vi "TTM 4He Press to Temp.vi"(1 "4He Vapor Pressure (torr)":dbl format="%.3f") -> (0 "4He Temp (K)":dbl format="%.3f")   [LabVIEW 2019]
panel:
  # "ITS-90 valid only from 1.25K to 2.17K"
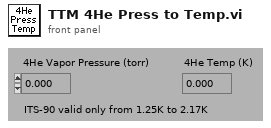
[diagram p1: front panel]
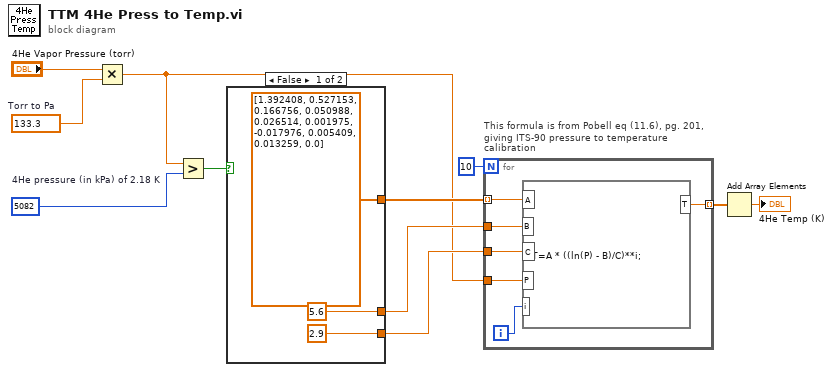
[diagram p0: block diagram]
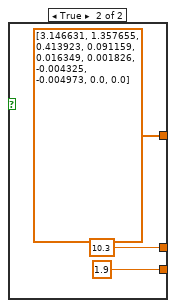
[diagram p2: hidden frame]
diagram:
  w2 = 133.3  # Torr to Pa
  w1 = 5082  # 4He pressure (in kPa) of 2.18 K
  n1 = Multiply(x="4He Vapor Pressure (torr)", y=w2) -> (x*y=w4:dbl)
  n2 = Greater?(x=w4, y=w1) -> (0:w8:bool)
  n3 = case shown="False" w8 {
    tunnel: [dbl[] [1.392408, 0.527153, 0.166756, 0.050988, 0.026514, 0.001975, -0.017976, 0.005409, 0.013259, 0.0] dbl[] [3.146631, 1.357655, 0.413923, 0.091159, 0.016349, 0.001826, -0.004325, -0.004973, 0.0, 0.0]] -> w7
    tunnel: [5.6 10.3] -> w6
    tunnel: [2.9 1.9] -> w5
    frame False {
    }
    frame True {
    }
  }
  n4 = for "This formula is from Pobell eq (11.6), pg. 201, giving ITS-90 pressure to temperature calibration" {
    N: 10 -> [_]
    tunnel: [w23] -> w11 mode=indexing
    tunnel: w4 -> [w22]
    tunnel: w7 -> [w21] mode=indexing
    tunnel: w6 -> [w20]
    tunnel: w5 -> [w19]
    i -> [w18]
    n5 = formula code="T=A * ((ln(P) - B)/C)**i;"("A"=w21, "B"=w20, "C"=w19, "P"=w22, "i"=w18) -> ("T"=w23:dbl)
  }
  n6 = Add Array Elements(numeric array=w11) -> (sum=→"4He Temp (K)":dbl)
